vi "Read ServerName.vi"(8 "error in (no error)":errorcluster, 11 "DIMActor in":refnum<class "DIMActor.lvclass">) -> (0 "error out":errorcluster, 2 "ServerName":string, 3 "DIMActor out":refnum<class "DIMActor.lvclass">)   [LabVIEW 2012, in "DIMActor.lvlib" / "DIMActor.lvclass"]
doc: "Read DIM server name."
uses:
  DIMActor.lvclass
  DIMActor.lvclass/DIMActor.ctl
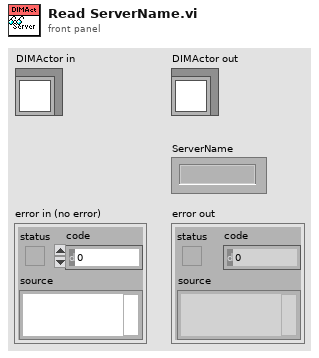
[diagram p1: front panel]
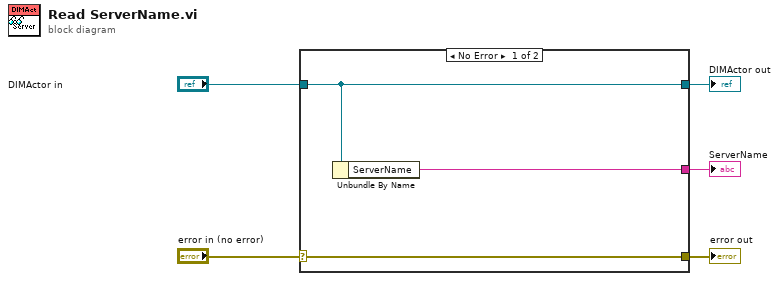
[diagram p0: block diagram]
diagram:
  n1 = case shown="No Error" "error in (no error)" {
    selector: "error in (no error)" -> [w8 w9]
    tunnel: [w8 w9] -> w4
    tunnel: [w7 w10] -> w2
    tunnel: "DIMActor in" -> [w7 w10]
    tunnel: [w6 _] -> w1
    frame No Error {
      n2 = Unbundle By Name(w7) -> ("ServerName"=w6:string)
    }
    frame Error {
    }
  }
  "error out" <- w4
  "DIMActor out" <- w2
  "ServerName" <- w1
